vi "Begin.vi"(8 "error in":errorcluster) -> (0 "error out":errorcluster)   [LabVIEW 2017]
doc: "Called before other user functions, this VI is expected to open initial I/O refnums, load in file data, and do all program initialization. Notice that the <B>error out</B> terminal is simply used for data flow. Wiring it to other structures or subVIs ensures that this VI runs first."
uses:
  <vilib>/Rock Robotics/WPI/DriverStation/WPI_DriverStationRobotMode2.ctl
  <vilib>/Rock Robotics/WPI/Joystick/WPI_JoystickDeviceEnum.ctl
  Public/Documents/Cross The Road Electronics/Phoenix-LabVIEW/Motor Controller/Controls/CTRE_Phoenix_MotorControl_ControlMode.ctl
  <vilib>/Rock Robotics/WPI/Solenoid/WPI_SolenoidChannel.ctl
  Public/Documents/Cross The Road Electronics/Phoenix-LabVIEW/Motor Controller/Controls/CTRE_Phoenix_MotorControl_FeedbackDevice.ctl
  <vilib>/Rock Robotics/SystemInterfaces/AI/FPGA_AIChannel.ctl
  <vilib>/Rock Robotics/WPI/SafetyOutput/WPI_SafetyOutputConfigMenu.ctl
  Robot Global Data.vi
  <vilib>/Rock Robotics/Network Tables/NT Write String Array.vi
  <vilib>/Rock Robotics/WPI/Solenoid/WPI_SolenoidOpenDouble.vi
  <vilib>/Rock Robotics/WPI/Utilities/WPI_GetSetVariantRefNum.vi
  <vilib>/Rock Robotics/WPI/RobotDrive/WPI_RobotDriveOpen2MotorWithExistingMotors.vi
panel:
  in  "Percent Deadband":dbl
  in  "Ramp Rate\nSeconds Closed":dbl
  in  "Ramp Rate\nSecond Open":dbl
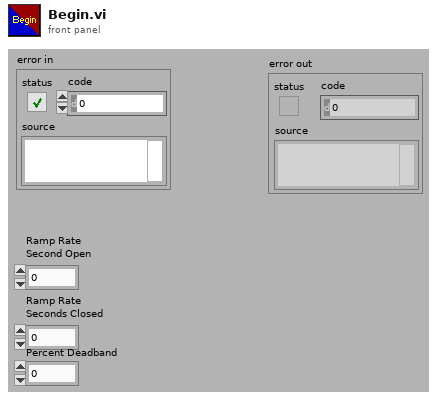
[diagram p1: front panel]
types:
  T1 = typedef "WPI_SafetyOutputConfigMenu.ctl" = enum16{"Enable", "Disable"}
  T2 = typedef "FPGA_AIChannel.ctl" = enum8{"AI 0", "AI 1", "AI 2", "AI 3", "AI MXP 0", "AI MXP 1", "AI MXP 2", "AI MXP 3", "Invalid"}
  T3 = typedef "CTRE_Phoenix_MotorControl_FeedbackDevice.ctl" = i8
  T4 = typedef "WPI_SolenoidChannel.ctl" = enum8{"Solenoid 0", "Solenoid 1", "Solenoid 2", "Solenoid 3", "Solenoid 4", "Solenoid 5", "Solenoid 6", "Solenoid 7", "Invalid"}
  T5 = typedef "WPI_JoystickDeviceEnum.ctl" = enum16{"USB 0", "USB 1", "USB 2", "USB 3", "USB 4", "USB 5"}
  T6 = typedef "CTRE_Phoenix_MotorControl_ControlMode.ctl" = u16
  T7 = typedef "WPI_DriverStationRobotMode2.ctl" = enum16{"Autonomous Disabled", "Autonomous Enabled", "Teleop Disabled", "Teleop Enabled", "Disconnected", "Finish", "Test Disabled", "Test Enabled", "Emergency Stopped"}
  T8 = typedef "WPI_SolenoidDevRef.ctl" = cluster{"DevStatus":errorcluster, "Pneumatics Control Module":u8, "Forward Solenoid Channel":T4, "Reverse Solenoid Channel":T4}
  T9 = typedef "WPI_CompressorDevRef.ctl" = cluster{"DevStatus":errorcluster, "Pneumatics Control Module":u8}
  T10 = typedef "WPI_MotorControlDeviceRef.ctl" = cluster{"DeviceStatus":errorcluster, "Type":T11, "PWM":cluster{"PWM Channel":T12, "DeadBand":T13}, "CAN":cluster{"Device Number":u8, "SetOutput VI Ref":variant, "GetOutput VI Ref":variant, "Enable VI Ref":variant, "Disable VI Ref":variant, "Data":variant}, "Invert":bool, "DIO PWM":cluster{"PWM \"Enable\" Channel":T12, "DIOChannel":T14, "PWM Rate":dbl}}
  T11 = typedef "WPI_MotorControlType.ctl" = enum16{"PWM", "CAN", "DIO PWM"}
  T12 = typedef "FPGA_DIOPWMChannel.ctl" = enum8{"PWM 0", "PWM 1", "PWM 2", "PWM 3", "PWM 4", "PWM 5", "PWM 6", "PWM 7", "PWM 8", "PWM 9", "PWM MXP 0", "PWM MXP 1", "PWM MXP 2", "PWM MXP 3", "PWM MXP 4", "PWM MXP 5", "PWM MXP 6", "PWM MXP 7", "PWM MXP 8", "PWM MXP 9", "Invalid"}
  T13 = typedef "WPI_PWMDeadband.ctl" = cluster{"Name":string, "maxPositivePwm":i32, "minPositivePwm":i32, "centerPwm":i32, "maxNegativePwm":i32, "minNegativePwm":i32, "angularRange":u16}
  T14 = typedef "FPGA_DIOChannel.ctl" = enum8{"DIO 0", "DIO 1", "DIO 2", "DIO 3", "DIO 4", "DIO 5", "DIO 6", "DIO 7", "DIO 8", "DIO 9", "DIO MXP 0", "DIO MXP 1", "DIO MXP 2", "DIO MXP 3", "DIO MXP 4", "DIO MXP 5", "DIO MXP 6", "DIO MXP 7", "DIO MXP 8", "DIO MXP 9", "DIO MXP 10", "DIO MXP 11", "DIO MXP 12", "DIO MXP 13", "DIO MXP 14", "DIO MXP 15", "SPI Port CS1", "SPI Port CS2", "SPI Port CS3", "SPI Port MISO", "SPI Port MOSI", "Invalid"}
  T15 = typedef "WPI_JoystickDevRef.ctl" = cluster{"Device":T5}
  T16 = typedef "WPI_AnalogChannelDevRef.ctl" = cluster{"DevStatus":errorcluster, "Analog Channel":T2}
  T17 = typedef "WPI_RobotDriveDevRef.ctl" = cluster{"DevStatus":errorcluster, "Motors[]":T10[], "Square Inputs":bool, "Max Output":dbl}
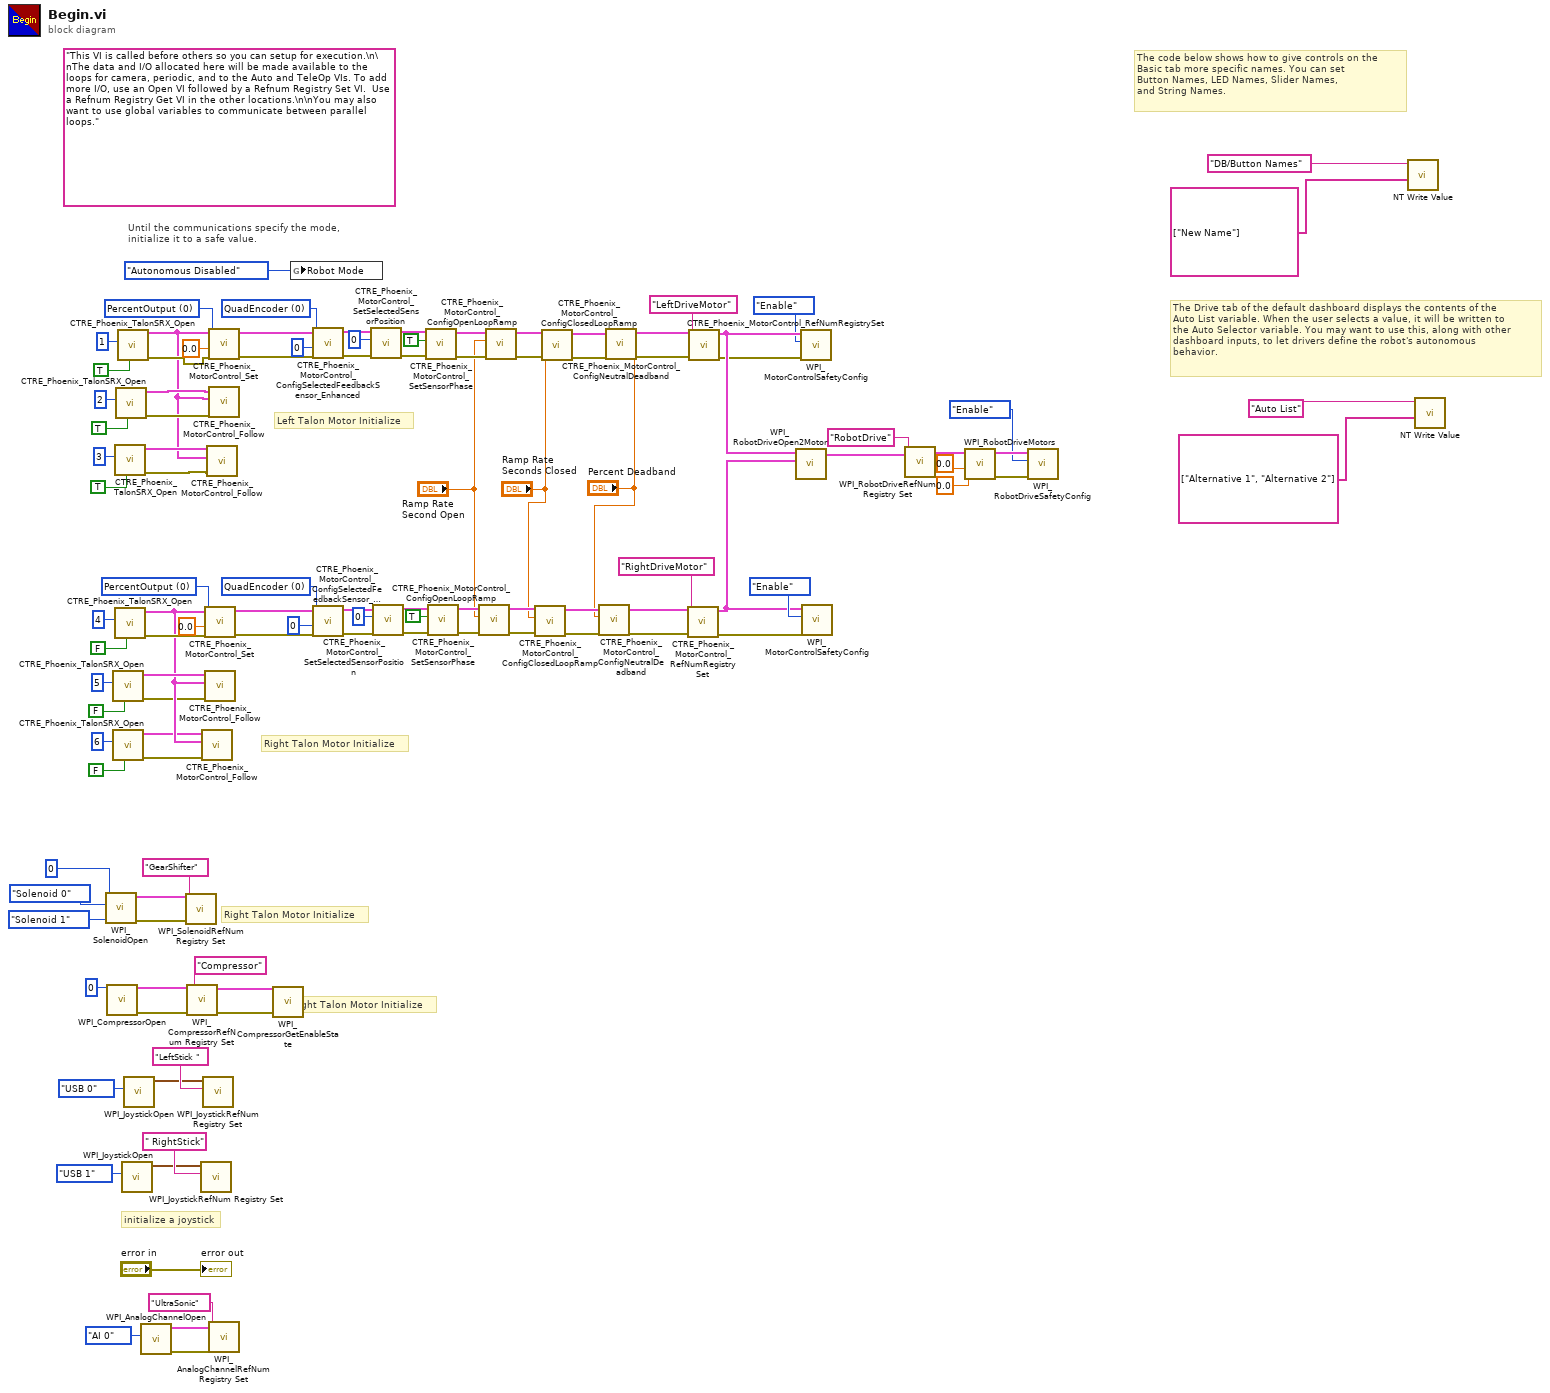
[diagram p0: block diagram]
diagram:
  w58 = T3 0 items=["None"=-1, "QuadEncoder"=0, "Analog"=2, "Tachometer"=4, "Pulse Width Encoded Position"=8, "Sensor Sum (S0 + S1)"=9, "Sensor Difference (D0 - D1)"=10, "Remote Source 0"=11, "Remote Source 1"=12, "Software Emulated"=15] ("Feedback Device")
  w60 = T3 0 items=["None"=-1, "QuadEncoder"=0, "Analog"=2, "Tachometer"=4, "Pulse Width Encoded Position"=8, "Sensor Sum (S0 + S1)"=9, "Sensor Difference (D0 - D1)"=10, "Remote Source 0"=11, "Remote Source 1"=12, "Software Emulated"=15] ("Feedback Device")
  w96 = T6 0 items=["PercentOutput"=0, "Position"=1, "Velocity"=2, "Current"=3, "Follower"=5, "MotionProfile"=6, "MotionMagic"=7, "MotionMagicArc"=8, "MotionProfileArc"=10, "Disabled"=15] ("Control Mode")
  w100 = T6 0 items=["PercentOutput"=0, "Position"=1, "Velocity"=2, "Current"=3, "Follower"=5, "MotionProfile"=6, "MotionMagic"=7, "MotionMagicArc"=8, "MotionProfileArc"=10, "Disabled"=15] ("Control Mode")
  (unwired) "This VI is called before others so you can setup for execution.\n\nThe data and I/O allocated here will be made available to the loops for camera, periodic, and to the Auto and TeleOp VIs. To add more I/O, use an Open VI followed by a Refnum Registry Set VI.  Use a Refnum Registry Get VI in the other locations.\n\nYou may also want to use global variables to communicate between parallel loops."
  # "Right Talon Motor Initialize"
  # "Right Talon Motor Initialize"
  # "Right Talon Motor Initialize"
  # "Left Talon Motor Initialize"
  # "The Drive tab of the default dashboard displays the contents of the\nAuto List variable. When the user selects a value, it will be written to\nthe Auto Selector variable. You may want to use this, along with other\ndashboard inputs, to let drivers define the robot's autonomous\nbehavior."
  # "The code below shows how to give controls on the\nBasic tab more specific names. You can set\nButton Names, LED Names, Slider Names,\nand String Names."
  # "initialize a joystick"
  # "Until the communications specify the mode,\ninitialize it to a safe value."
  n1 = call-poly <vilib>:"WPI_SolenoidOpen.vi"("Reverse Solenoid Channel"=WPI_SolenoidChannel."Solenoid 1", "Forward Solenoid Channel"=WPI_SolenoidChannel."Solenoid 0" ("Solenoid Channel"), "Pneumatics Control Module (0)"=u8 0) -> ("error out"=w70:errorcluster, "SolenoidDevRef"=w71:T8)  [unwired: 7 in]
  n2 = call <vilib>:"WPI_CompressorOpen.vi"("Pneumatics Control Module (0)"=u8 0) -> ("CompressorDevRef"=w68:T9, "error out"=w67:errorcluster)  [unwired: 13 in]
  n3 = call "CTRE_Phoenix_TalonSRX_Open.vi"("Invert"=FALSE, "Device Number"=u8 5) -> ("error out"=w38:errorcluster, "CAN Talon SRX Ref"=w42:T10)  [unwired: 8 in]
  n4 = call "CTRE_Phoenix_TalonSRX_Open.vi"("Invert"=FALSE, "Device Number"=u8 6) -> ("error out"=w39:errorcluster, "CAN Talon SRX Ref"=w40:T10)  [unwired: 8 in]
  n5 = call "CTRE_Phoenix_TalonSRX_Open.vi"("Invert"=TRUE, "Device Number"=u8 3) -> ("error out"=w33:errorcluster, "CAN Talon SRX Ref"=w36:T10)  [unwired: 8 in]
  n6 = call "CTRE_Phoenix_TalonSRX_Open.vi"("Invert"=FALSE, "Device Number"=u8 4) -> ("error out"=w75:errorcluster, "CAN Talon SRX Ref"=w41:T10)  [unwired: 8 in]
  n7 = call "CTRE_Phoenix_TalonSRX_Open.vi"("Invert"=TRUE, "Device Number"=u8 2) -> ("error out"=w37:errorcluster, "CAN Talon SRX Ref"=w35:T10)  [unwired: 8 in]
  n8 = call "CTRE_Phoenix_TalonSRX_Open.vi"("Invert"=TRUE, "Device Number"=u8 1) -> ("error out"=w76:errorcluster, "CAN Talon SRX Ref"=w34:T10)  [unwired: 8 in]
  n9 = call <vilib>:"WPI_JoystickOpen.vi"("JoystickDevice"=WPI_JoystickDeviceEnum."USB 1") -> ("JoystickDevRef"=w109:T15)  [unwired: 10 in]
  n10 = call <vilib>:"WPI_JoystickOpen.vi"("JoystickDevice"=WPI_JoystickDeviceEnum."USB 0") -> ("JoystickDevRef"=w80:T15)  [unwired: 10 in]
  n11 = call <vilib>:"WPI_AnalogChannelOpen.vi"("Analog Channel"=FPGA_AIChannel."AI 0") -> ("error out"=w30:errorcluster, "AIDeviceRef"=w31:T16)  [unwired: 9 in]
  n12 = call <vilib>:"WPI_SolenoidRefNum Registry Set.vi"("error in (no error)"=w70, "refnum name"="GearShifter", "SolenoidDevRef"=w71) -> ()  [unwired: 7 in, 2 out]
  n13 = call <vilib>:"WPI_CompressorRefNum Registry Set.vi"("error in (no error)"=w67, "refnum name"="Compressor", "CompressorDevRef"=w68) -> ("error out"=w65:errorcluster, "CompressorDevRef"=w66:T9)  [unwired: 7 in]
  n14 = call <vilib>:"WPI_JoystickRefNum Registry Set.vi"("refnum name"=" RightStick", "JoystickDevRef"=w109) -> ()  [unwired: 8 in, 2 out]
  n15 = call "CTRE_Phoenix_MotorControl_Follow.vi"("error in (no error)"=w39, "Master Controller to Follow"=w41, "PhoenixMotorControlDevRef"=w40) -> ()  [unwired: 7 in, 2 out]
  n16 = call <vilib>:"WPI_JoystickRefNum Registry Set.vi"("refnum name"="LeftStick ", "JoystickDevRef"=w80) -> ()  [unwired: 8 in, 2 out]
  n17 = call "CTRE_Phoenix_MotorControl_Set.vi"("error in (no error)"=w75, "Output"=0.0, "Control Mode"=w96, "PhoenixMotorControlDevRef"=w41) -> ("error out"=w55:errorcluster, "PhoenixMotorControlDevRef"=w56:T10)  [unwired: 6 in]
  n18 = call "CTRE_Phoenix_MotorControl_Follow.vi"("error in (no error)"=w38, "Master Controller to Follow"=w41, "PhoenixMotorControlDevRef"=w42) -> ()  [unwired: 7 in, 2 out]
  n19 = call "CTRE_Phoenix_MotorControl_Follow.vi"("error in (no error)"=w33, "Master Controller to Follow"=w34, "PhoenixMotorControlDevRef"=w36) -> ()  [unwired: 7 in, 2 out]
  n20 = call "CTRE_Phoenix_MotorControl_Set.vi"("error in (no error)"=w76, "Output"=0.0, "Control Mode"=w100, "PhoenixMotorControlDevRef"=w34) -> ("error out"=w61:errorcluster, "PhoenixMotorControlDevRef"=w62:T10)  [unwired: 6 in]
  n21 = call "CTRE_Phoenix_MotorControl_Follow.vi"("error in (no error)"=w37, "Master Controller to Follow"=w34, "PhoenixMotorControlDevRef"=w35) -> ()  [unwired: 7 in, 2 out]
  n22 = call <vilib>:"WPI_AnalogChannelRefNum Registry Set.vi"("error in (no error)"=w30, "refnum name"="UltraSonic", "AIDeviceRef"=w31) -> ()  [unwired: 7 in, 2 out]
  n23 = call <vilib>:"WPI_CompressorGetEnableState.vi"("error in (no error)"=w65, "CompressorDevRef"=w66) -> ()  [unwired: 6 in, 4 out]
  n24 = global write "Robot Global Data.vi" "Robot Mode"(WPI_DriverStationRobotMode2."Autonomous Disabled" ("Robot Mode")) -> ()
  n25 = call "CTRE_Phoenix_MotorControl_ConfigSelectedFeedbackSensor_Enhanced.vi"("error in (no error)"=w61, "pidLoopIdx"=0, "Feedback Device"=w60, "PhoenixMotorControlDevRef"=w62) -> ("error out"=w54:errorcluster, "PhoenixMotorControlDevRef"=w53:T10)  [unwired: 6 in]
  n26 = call "CTRE_Phoenix_MotorControl_ConfigSelectedFeedbackSensor_Enhanced.vi"("error in (no error)"=w55, "pidLoopIdx"=0, "Feedback Device"=w58, "PhoenixMotorControlDevRef"=w56) -> ("error out"=w50:errorcluster, "PhoenixMotorControlDevRef"=w49:T10)  [unwired: 6 in]
  n27 = call "CTRE_Phoenix_MotorControl_SetSelectedSensorPosition.vi"("error in (no error)"=w54, "New Sensor Position"=0, "PhoenixMotorControlDevRef"=w53) -> ("error out"=w47:errorcluster, "PhoenixMotorControlDevRef"=w48:T10)  [unwired: 7 in]
  n28 = call "CTRE_Phoenix_MotorControl_SetSelectedSensorPosition.vi"("error in (no error)"=w50, "New Sensor Position"=0, "PhoenixMotorControlDevRef"=w49) -> ("error out"=w45:errorcluster, "PhoenixMotorControlDevRef"=w44:T10)  [unwired: 7 in]
  n29 = call "CTRE_Phoenix_MotorControl_SetSensorPhase.vi"("error in (no error)"=w47, "PhaseSensor"=TRUE, "PhoenixMotorControlDevRef"=w48) -> ("error out"=w15:errorcluster, "PhoenixMotorControlDevRef"=w19:T10)  [unwired: 7 in]
  n30 = call "CTRE_Phoenix_MotorControl_SetSensorPhase.vi"("error in (no error)"=w45, "PhaseSensor"=TRUE, "PhoenixMotorControlDevRef"=w44) -> ("error out"=w6:errorcluster, "PhoenixMotorControlDevRef"=w7:T10)  [unwired: 7 in]
  n31 = call "CTRE_Phoenix_MotorControl_ConfigOpenLoopRamp.vi"("error in (no error)"=w6, "secondsFromNeutralToFull"="Ramp Rate\nSecond Open", "PhoenixMotorControlDevRef"=w7) -> ("error out"=w9:errorcluster, "PhoenixMotorControlDevRef"=w11:T10)  [unwired: 7 in]
  n32 = call "CTRE_Phoenix_MotorControl_ConfigOpenLoopRamp.vi"("error in (no error)"=w15, "secondsFromNeutralToFull"="Ramp Rate\nSecond Open", "PhoenixMotorControlDevRef"=w19) -> ("error out"=w14:errorcluster, "PhoenixMotorControlDevRef"=w18:T10)  [unwired: 7 in]
  n33 = call "CTRE_Phoenix_MotorControl_ConfigClosedLoopRamp.vi"("error in (no error)"=w9, "secondsFromNeutralToFull"="Ramp Rate\nSeconds Closed", "PhoenixMotorControlDevRef"=w11) -> ("error out"=w8:errorcluster, "PhoenixMotorControlDevRef"=w10:T10)  [unwired: 7 in]
  n34 = call "CTRE_Phoenix_MotorControl_ConfigClosedLoopRamp.vi"("error in (no error)"=w14, "secondsFromNeutralToFull"="Ramp Rate\nSeconds Closed", "PhoenixMotorControlDevRef"=w18) -> ("error out"=w13:errorcluster, "PhoenixMotorControlDevRef"=w17:T10)  [unwired: 7 in]
  n35 = call "CTRE_Phoenix_MotorControl_ConfigNeutralDeadband.vi"("error in (no error)"=w8, "Percent Deadband"="Percent Deadband", "PhoenixMotorControlDevRef"=w10) -> ("error out"=w4:errorcluster, "PhoenixMotorControlDevRef"=w5:T10)  [unwired: 7 in]
  n36 = call "CTRE_Phoenix_MotorControl_ConfigNeutralDeadband.vi"("error in (no error)"=w13, "Percent Deadband"="Percent Deadband", "PhoenixMotorControlDevRef"=w17) -> ("error out"=w12:errorcluster, "PhoenixMotorControlDevRef"=w16:T10)  [unwired: 7 in]
  n37 = call "CTRE_Phoenix_MotorControl_RefNumRegistrySet.vi"("error in (no error)"=w4, "refnum name"="RightDriveMotor", "PhoenixMotorControlDevRef"=w5) -> ("error out"=w22:errorcluster, "PhoenixMotorControlDevRef"=w25:T10)  [unwired: 7 in]
  n38 = call "CTRE_Phoenix_MotorControl_RefNumRegistrySet.vi"("error in (no error)"=w12, "refnum name"="LeftDriveMotor", "PhoenixMotorControlDevRef"=w16) -> ("error out"=w21:errorcluster, "PhoenixMotorControlDevRef"=w28:T10)  [unwired: 7 in]
  n39 = call-poly <vilib>:"WPI_RobotDriveOpen2Motor.vi"("Right Motor Dev Ref"=w25, "Left Motor Dev Ref"=w28) -> ("RobotDriveDevRef"=w86:T17)  [unwired: 8 in, 1 out]
  n40 = call <vilib>:"WPI_MotorControlSafetyConfig.vi"("error in (no error)"=w21, "mode"=WPI_SafetyOutputConfigMenu."Enable", "MotorControlDevRef"=w28) -> ()  [unwired: 7 in, 2 out]
  n41 = call <vilib>:"WPI_MotorControlSafetyConfig.vi"("error in (no error)"=w22, "mode"=WPI_SafetyOutputConfigMenu."Enable", "MotorControlDevRef"=w25) -> ()  [unwired: 7 in, 2 out]
  n42 = call <vilib>:"WPI_RobotDriveRefNum Registry Set.vi"("refnum name"="RobotDrive", "RobotDriveDevRef"=w86) -> ("RobotDriveDevRef"=w84:T17)  [unwired: 8 in, 1 out]
  n43 = call <vilib>:"WPI_RobotDriveMotors.vi"("RightSpeed"=0.0, "LeftSpeed"=0.0, "RobotDriveDevRef"=w84) -> ("error out"=w23:errorcluster, "RobotDriveDevRef"=w24:T17)  [unwired: 6 in, 1 out]
  n44 = call <vilib>:"WPI_RobotDriveSafetyConfig.vi"("error in (no error)"=w23, "mode"=WPI_SafetyOutputConfigMenu."Enable", "RobotDriveDevRef"=w24) -> ()  [unwired: 7 in, 2 out]
  n45 = call-poly <vilib>:"NT Write Value.vi"("String Array"=string[] ["New Name"], "Name"="DB/Button Names") -> ()  [unwired: 9 in, 1 out]
  n46 = call-poly <vilib>:"NT Write Value.vi"("String Array"=string[] ["Alternative 1", "Alternative 2"], "Name"="Auto List") -> ()  [unwired: 9 in, 1 out]
  "error out" <- "error in"
